vi "retroreflectivetapesample2.vi"(0 "Color Mode (Color Threshold 1)":u16(ring) items=["RGB", "HSL", "HSV", "HSI"], 1 "Red or Hue Range (Color Threshold 1)":cluster{"Lower value":i32, "Upper value":i32}={"Lower value"=0, "Upper value"=160}, 2 "Green or Sat Range (Color Threshold 1)":cluster{"Lower value":i32, "Upper value":i32}={"Lower value"=127, "Upper value"=199}, 3 "Blue or Luma or Val or Inten Range (Color Threshold 1)":cluster{"Lower value":i32, "Upper value":i32}={"Lower value"=66, "Upper value"=182}, 4 "Pixel Measurements (Particle Analysis 1)":i32[](array[ring])=[0, 1, 4, 5, 6, 7, 16, 17, 35] items=["Center of Mass X", "Center of Mass Y", "First Pixel X", "First Pixel Y", "Bounding Rect Left", "Bounding Rect Top", "Bounding Rect Right", "Bounding Rect Bottom", "Max Feret Diameter Start X", "Max Feret Diameter Start Y", "Max Feret Diameter End X", "Max Feret Diameter End Y", "Max Horiz. Segment Length Left", "Max Horiz. Segment Length Right", "Max Horiz. Segment Length Row", "-", "Bounding Rect Width", "Bounding Rect Height", "Bounding Rect Diagonal", "Perimeter", "Convex Hull Perimeter", "Holes' Perimeter", "Max Feret Diameter", "Equivalent Ellipse Major Axis", "Equivalent Ellipse Minor Axis", "Equivalent Ellipse Minor Axis (Feret)", "Equivalent Rect Long Side", "Equivalent Rect Short Side", "Equivalent Rect Diagonal", "Equivalent Rect Short Side (Feret)", "Average Horiz. Segment Length", "Average Vert. Segment Length", "Hydraulic Radius", "Waddel Disk Diameter", "-", "Area", "Holes' Area", "Particle & Holes' Area", "Convex Hull Area", "Image Area", "-", "Number of Holes", "Number of Horiz. Segments", "Number of Vert. Segments", "-", "Orientation", "Max Feret Diameter Orientation", "-", "% Area/Image Area", "% Area/(Particle & Holes' Area)", "Ratio of Equivalent Ellipse Axes", "Ratio of Equivalent Rect Sides", "-", "Elongation Factor", "Compactness Factor", "Heywood Circularity Factor", "Type Factor", "-", "Sum X", "Sum Y", "Sum XX", "Sum XY", "Sum YY", "Sum XXX", "Sum XXY", "Sum XYY", "Sum YYY", "-", "Moment of Inertia XX", "Moment of Inertia XY", "Moment of Inertia YY", "Moment of Inertia XXX", "Moment of Inertia XXY", "Moment of Inertia XYY", "Moment of Inertia YYY", "Norm. Moment of Inertia XX", "Norm. Moment of Inertia XY", "Norm. Moment of Inertia YY", "Norm. Moment of Inertia XXX", "Norm. Moment of Inertia XXY", "Norm. Moment of Inertia XYY", "Norm. Moment of Inertia YYY", "Hu Moment 1", "Hu Moment 2", "Hu Moment 3", "Hu Moment 4", "Hu Moment 5", "Hu Moment 6", "Hu Moment 7"], 5 "Real-World Measurements (Particle Analysis 1)":i32[](array[ring]) items=["Center of Mass X", "Center of Mass Y", "First Pixel X", "First Pixel Y", "Bounding Rect Left", "Bounding Rect Top", "Bounding Rect Right", "Bounding Rect Bottom", "Max Feret Diameter Start X", "Max Feret Diameter Start Y", "Max Feret Diameter End X", "Max Feret Diameter End Y", "Max Horiz. Segment Length Left", "Max Horiz. Segment Length Right", "Max Horiz. Segment Length Row", "-", "Bounding Rect Width", "Bounding Rect Height", "Bounding Rect Diagonal", "Perimeter", "Convex Hull Perimeter", "Holes' Perimeter", "Max Feret Diameter", "Equivalent Ellipse Major Axis", "Equivalent Ellipse Minor Axis", "Equivalent Ellipse Minor Axis (Feret)", "Equivalent Rect Long Side", "Equivalent Rect Short Side", "Equivalent Rect Diagonal", "Equivalent Rect Short Side (Feret)", "Average Horiz. Segment Length", "Average Vert. Segment Length", "Hydraulic Radius", "Waddel Disk Diameter", "-", "Area", "Holes' Area", "Particle & Holes' Area", "Convex Hull Area", "Image Area", "-", "Number of Holes", "Number of Horiz. Segments", "Number of Vert. Segments", "-", "Orientation", "Max Feret Diameter Orientation", "-", "% Area/Image Area", "% Area/(Particle & Holes' Area)", "Ratio of Equivalent Ellipse Axes", "Ratio of Equivalent Rect Sides", "-", "Elongation Factor", "Compactness Factor", "Heywood Circularity Factor", "Type Factor", "-", "Sum X", "Sum Y", "Sum XX", "Sum XY", "Sum YY", "Sum XXX", "Sum XXY", "Sum XYY", "Sum YYY", "-", "Moment of Inertia XX", "Moment of Inertia XY", "Moment of Inertia YY", "Moment of Inertia XXX", "Moment of Inertia XXY", "Moment of Inertia XYY", "Moment of Inertia YYY", "Norm. Moment of Inertia XX", "Norm. Moment of Inertia XY", "Norm. Moment of Inertia YY", "Norm. Moment of Inertia XXX", "Norm. Moment of Inertia XXY", "Norm. Moment of Inertia XYY", "Norm. Moment of Inertia YYY", "Hu Moment 1", "Hu Moment 2", "Hu Moment 3", "Hu Moment 4", "Hu Moment 5", "Hu Moment 6", "Hu Moment 7"], 7 "error in":errorcluster) -> (20 "Number of Particles (Particle Analysis 1)":i32, 21 "Particle Measurements (Pixels) (Particle Analysis 1)":dbl[][](array[numeric]) format="%.2f", 22 "Particle Measurements (Real-World) (Particle Analysis 1)":dbl[][](array[numeric]) format="%.2f", 27 "error out":errorcluster)   [LabVIEW 2015]
uses:
  <vilib>/vision/NI_Vision_Development_Module.lvlib
panel:
  out "Arm Movement":dbl
  out "Rotation":dbl
  out "Image Out":T1(plugin-control)
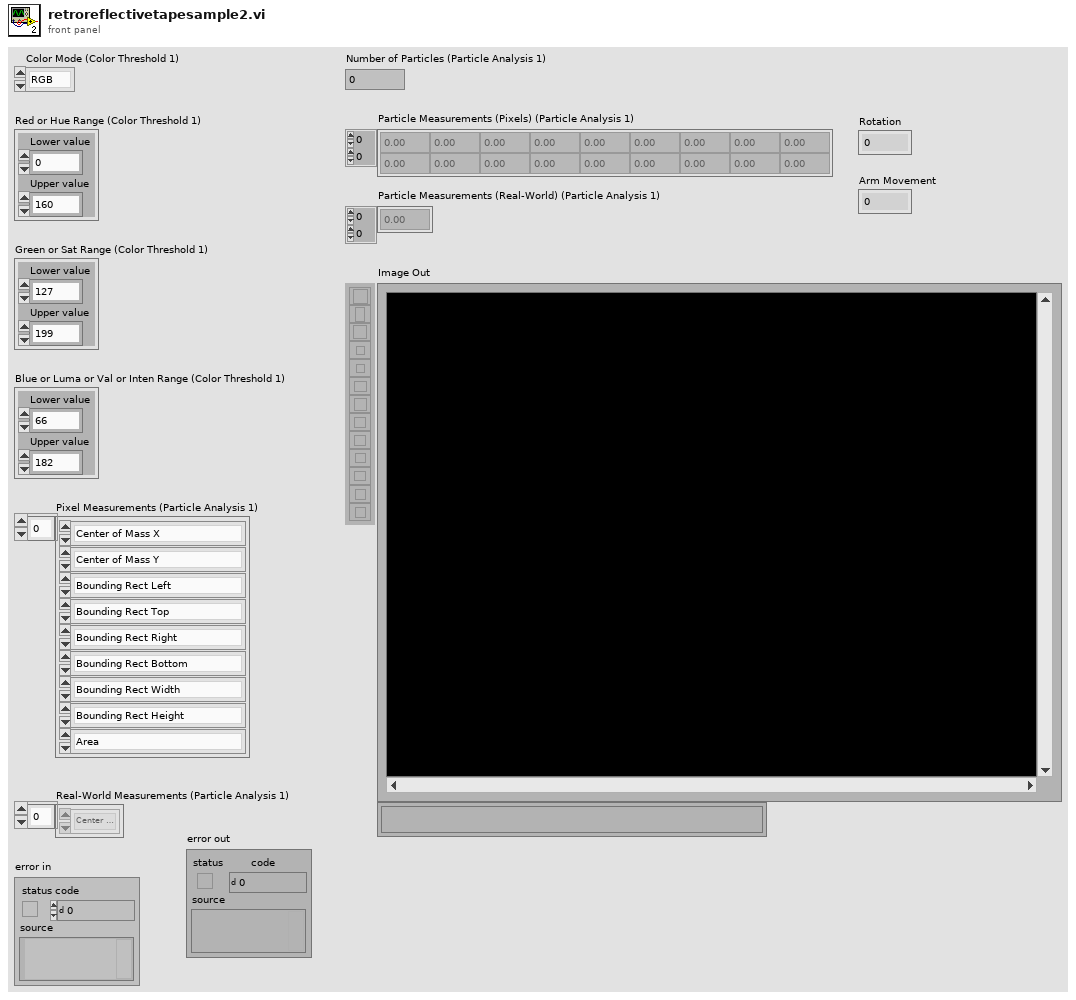
[diagram p1: front panel]
types:
  T1 = typedef "IMAQ Image.ctl" = refnum<image>
  T2 = enum32{"AutoM", "Close", "Dilate", "Erode", "Gradient", "Gradient out", "Gradient in", "Hit miss", "Open", "PClose", "POpen", "Thick", "Thin"}
  T3 = cluster{"Measurement Parameter":i32, "Range Lower Value":dbl, "Range Upper Value":dbl, "Range":bool, "Measurement Type":bool}[]
  T4 = typedef "Image Type" = u32
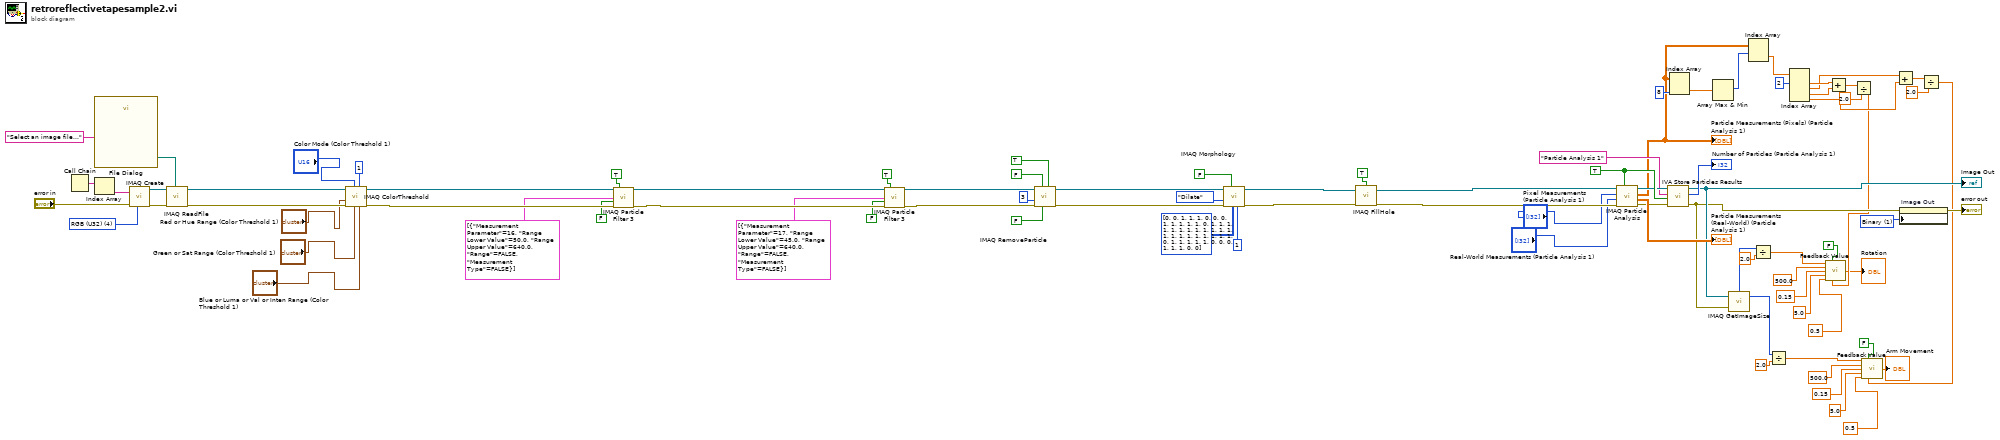
[diagram p0: block diagram]
diagram:
  w37 = u32 1 items=["Grayscale", "Binary", "Gradient", "Rainbow", "Temperature", "User Defined", "Binary 16 Bit", "Gradient 16 Bit", "Rainbow 16 Bit", "Temperature 16 Bit", "User Defined 16 Bit"] ("Palette Type")
  w43 = TRUE ("Connectivity 4/8 (8)")
  w80 = T4 4 items=["Grayscale (U8)", "Grayscale (I16)", "Grayscale (SGL)", "Complex (CSG)", "RGB (U32)", "HSL (U32)", "RGB (U64)", "Grayscale (U16)"] ("Image Type")
  n1 = Call Chain() -> (call chain=w84:string[])
  n2 = Index Array(array=w84) -> (element=w83:string)  [unwired: 1 in]
  n3 = call "File Dialog"("prompt"="Select an image file...") -> ("selected path"=w81:path)  [unwired: 6 in, 8 out]
  n4 = call "IMAQ Create"("Image Name"=w83, "Image Type"=w80, "error in (no error)"="error in") -> ("New Image"=w87:T1, "error out"=w86:errorcluster)  [unwired: 1 in, 1 out]
  n5 = call "IMAQ ReadFile"("File Path"=w81, "error in (no error)"=w86, "Image"=w87) -> ("error out"=w88:errorcluster, "Image Out"=w74:T1)  [unwired: 2 in, 5 out]
  n6 = call "IMAQ ColorThreshold"("Blue or Luma or Val or Inten Range"="Blue or Luma or Val or Inten Range (Color Threshold 1)", "Replace Value"=1, "Green or Sat Range"="Green or Sat Range (Color Threshold 1)", "Color Mode"="Color Mode (Color Threshold 1)", "error in (no error)"=w88, "Red or Hue Range"="Red or Hue Range (Color Threshold 1)", "Image Src"=w74) -> ("error out"=w73:errorcluster, "Image Dst Out"=w69:T1)  [unwired: 1 in, 2 out]
  n7 = call "IMAQ Particle Filter 3"("Image Src"=w69, "Connectivity 4/8 (8)"=TRUE, "Selection Values"=T3 [{"Measurement Parameter"=16, "Range Lower Value"=50.0, "Range Upper Value"=640.0, "Range"=FALSE, "Measurement Type"=FALSE}], "Keep/Remove Particles (F)"=FALSE ("Keep/Remove Particles"), "error in (no error)"=w73) -> ("Image Dst Out"=w64:T1, "error out"=w70:errorcluster)  [unwired: 4 in, 5 out]
  n8 = call "IMAQ Particle Filter 3"("Image Src"=w64, "Connectivity 4/8 (8)"=TRUE, "Selection Values"=T3 [{"Measurement Parameter"=17, "Range Lower Value"=45.0, "Range Upper Value"=640.0, "Range"=FALSE, "Measurement Type"=FALSE}], "Keep/Remove Particles (F)"=FALSE ("Keep/Remove Particles"), "error in (no error)"=w70) -> ("Image Dst Out"=w58:T1, "error out"=w65:errorcluster)  [unwired: 4 in, 5 out]
  n9 = call "IMAQ RemoveParticle"("Connectivity 4/8 (8)"=TRUE, "Low Pass/High Pass (Low)"=FALSE, "Square/Hexa (Square)"=FALSE, "error in (no error)"=w65, "Number of Erosion"=3, "Image Src"=w58) -> ("error out"=w57:errorcluster, "Image Dst Out"=w52:T1)  [unwired: 1 in, 3 out]
  n10 = call "IMAQ Morphology"("Number of iterations (1)"=1, "Structuring Element"=i32[][] [[0, 0, 1, 1, 1, 0, 0], [0, 1, 1, 1, 1, 1, 0], [1, 1, 1, 1, 1, 1, 1], [1, 1, 1, 1, 1, 1, 1], [1, 1, 1, 1, 1, 1, 1], [0, 1, 1, 1, 1, 1, 0], [0, 0, 1, 1, 1, 0, 0]], "Square/Hexa (Square)"=FALSE, "error in (no error)"=w57, "Operation"=T2."Dilate", "Image Src"=w52) -> ("error out"=w51:errorcluster, "Image Dst Out"=w49:T1)  [unwired: 1 in, 3 out]
  n11 = call "IMAQ FillHole"("error in (no error)"=w51, "Image Src"=w49, "Connectivity 4/8 (8)"=TRUE) -> ("error out"=w48:errorcluster, "Image Dst Out"=w44:T1)  [unwired: 1 in, 2 out]
  n12 = call "IMAQ Particle Analysis"("Connectivity 4/8 (8)"=w43, "error in (no error)"=w48, "Real-World Measurements"="Real-World Measurements (Particle Analysis 1)", "Pixel Measurements"="Pixel Measurements (Particle Analysis 1)", "Image"=w44) -> ("error out"=w40:errorcluster, "Particle Measurements (Real-World)"=→"Particle Measurements (Real-World) (Particle Analysis 1)":dbl[][], "Particle Measurements (Pixels)"=w26:dbl[][], "Image Out (duplicate)"=w42:T1)  [unwired: 3 out]
  "Particle Measurements (Pixels) (Particle Analysis 1)" <- w26
  n13 = call <vilib>:"IVA Store Particles Results.vi"("error in (no error)"=w40, "Connectivity 4/8 (8)"=w43, "Step Name"="Particle Analysis 1", "Image in"=w42) -> ("error out"=w35:errorcluster, "Number of Particles"=→"Number of Particles (Particle Analysis 1)":i32, "Image dup"=w36:T1)  [unwired: 5 out]
  "Image Out" <- w36
  n14 = Index Array(array=w26, index (col)=8 ("disabled index (col)")) -> (element=w27:dbl[])  [unwired: 1 in]
  n15 = Array Max & Min(array=w27) -> (max index (indices)=w25:i32)  [unwired: 3 out]
  n16 = call "IMAQ GetImageSize"("Image"=w36, "error in (no error)"=w35) -> ("Y Resolution"=w17:i32, "X Resolution"=w34:i32)  [unwired: 2 in, 1 out]
  n17 = Index Array(array=w26, index (row)=w25) -> (element=w24:dbl[])  [unwired: 1 in]
  n18 = Divide(x=w34, y=2.0) -> (x/y=w10:dbl)
  n19 = Divide(x=w17, y=2.0) -> (x/y=w3:dbl)
  n20 = Index Array(array=w24, index #1=2 ("index")) -> (element #1=w31:dbl, element #2=w19:dbl, element #3=w23:dbl, element #4=w20:dbl)  [unwired: 3 in]
  n21 = Add(x=w31, y=w23) -> (x+y=w30:dbl)
  n22 = Divide(x=w30, y=2.0) -> (x/y=w16:dbl)
  n23 = call "Feedback Value.vi"("Set Point"=w10, "Invert Rotation"=FALSE, "Divisor"=500.0, "Addend"=0.15, "Deadband"=5.0, "Maximum Amplitude"=0.5, "Current Value"=w16) -> ("Rotation"=→"Rotation":dbl)  [unwired: 8 in]
  n24 = Add(x=w19, y=w20) -> (x+y=w22:dbl)
  n25 = property on="Image Out" class="ImageControl"(error in=w35, "Palette:Palette Type"=w37) -> (error out=→"error out":errorcluster)  [unwired: 1 in, 1 out]
  n26 = Divide(x=w22, y=2.0) -> (x/y=w7:dbl)
  n27 = call "Feedback Value.vi"("Set Point"=w3, "Invert Rotation"=FALSE, "Divisor"=500.0, "Addend"=0.15, "Deadband"=5.0, "Maximum Amplitude"=0.5, "Current Value"=w7) -> ("Rotation"=→"Arm Movement":dbl)  [unwired: 8 in]
